vi "test Print Entry with Sub-Entries.vi"(11 "Test Case In":refnum<class "test Electronic Datasheet.lvclass">) -> (0 "error out":errorcluster, 3 "Test Case Out":refnum<class "test Electronic Datasheet.lvclass">)   [LabVIEW 2024, in "test Electronic Datasheet.lvclass"]
uses:
  test Electronic Datasheet.lvclass
  C:/Program Files/National Instruments/LabVIEW 2024/vi.lib/Astemes/LUnit/Test Case.lvclass
  <vilib>/Astemes/LUnit/Test Case.lvclass/Test Case.ctl
  2aee4a49-973f-4d4e-9175-22173d17c8e6.vi
  <vilib>/Astemes/LUnit/Append Pass Result.vi
  <vilib>/Astemes/LUnit/Append Fail Result.vi
  <vilib>/Astemes/LUnit/Describe Comparison.vi
  2aee4a49-973f-4d4e-9175-22173d17c8e6.vi/9c5d11cd-9439-4240-a1ee-d9baace9c924.vi
  <vilib>/Astemes/LUnit/Run In UI.vi
  <vilib>/Utility/error.llb/Clear Errors.vi
  Electronic Datasheet/utils/Electronic Datasheet_GetAttributes.vi
  <vilib>/Astemes/LUnit/Describe Variant.vi
  Electronic Datasheet/Electronic Datasheet.lvclass
  Core/OD Entry/OD Entry.lvclass
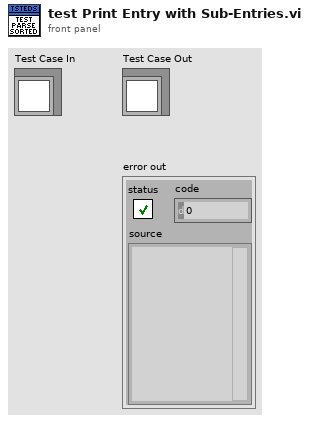
[diagram p1: front panel]
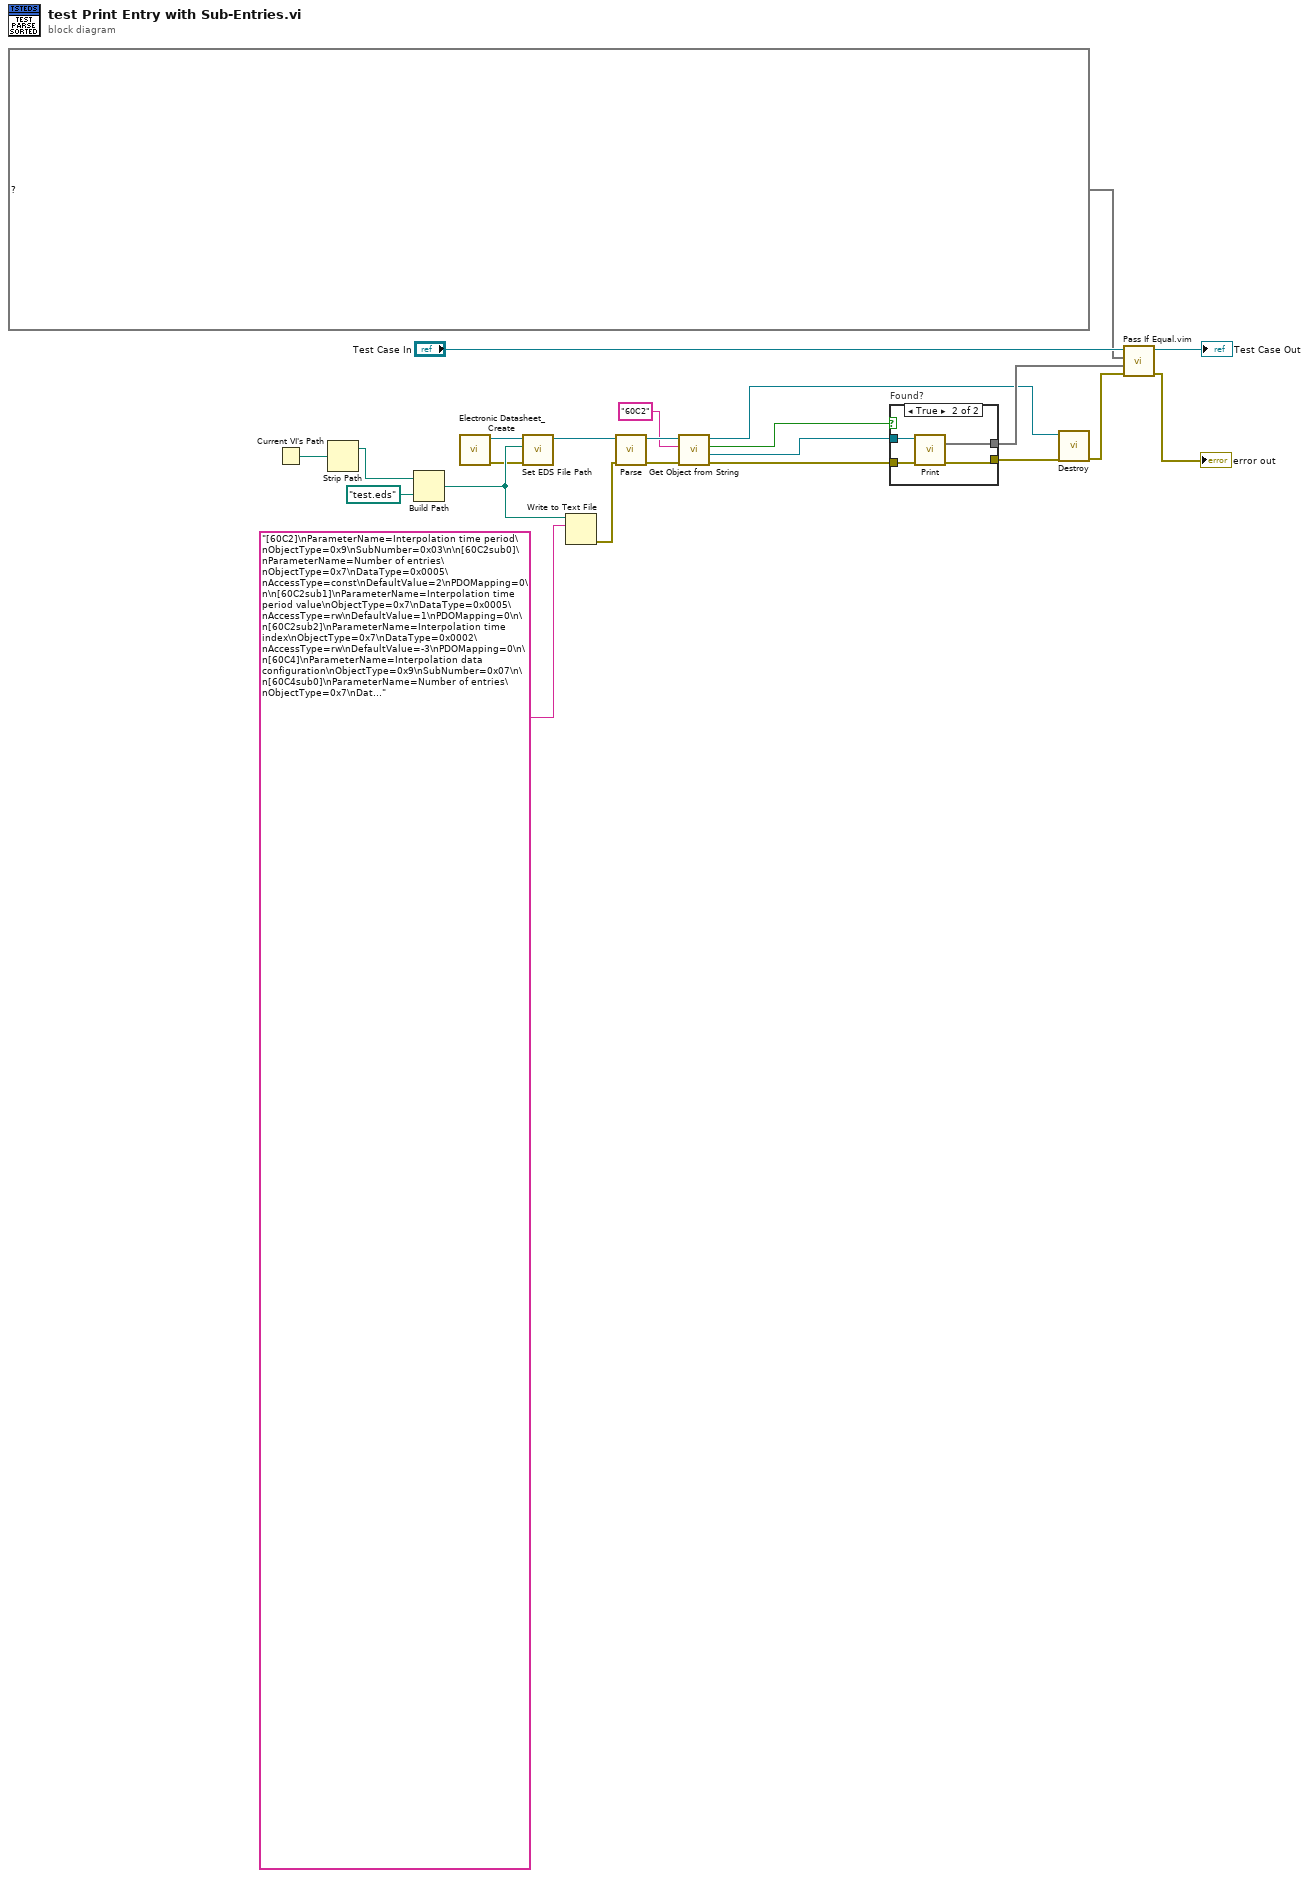
[diagram p0: block diagram]
diagram:
  n1 = Current VI's Path() -> (path=w19:path)
  n2 = Strip Path(path=w19) -> (stripped path=w15:path)  [unwired: 1 out]
  n3 = Build Path(base path=w15, name or relative path=path "test.eds") -> (appended path=w16:path)
  n4 = call "Electronic Datasheet_Create.vi"() -> ("Error Out"=w7:errorcluster, "reference out"=w8:refnum<class "Electronic Datasheet.lvclass">)  [unwired: 10 in]
  n5 = call "Set EDS File Path.vi"("error in"=w7, "EDS File Path"=w16, "reference in"=w8) -> ("reference out"=w20:refnum<class "Electronic Datasheet.lvclass">)  [unwired: 7 in, 1 out]
  n6 = Write to Text File(file (use dialog)=w16, text="[60C2]\nParameterName=Interpolation time period\nObjectType=0x9\nSubNumber=0x03\n\n[60C2sub0]\nParameterName=Number of entries\nObjectType=0x7\nDataType=0x0005\nAccessType=const\nDefaultValue=2\nPDOMapping=0\n\n[60C2sub1]\nParameterName=Interpolation time period value\nObjectType=0x7\nDataType=0x0005\nAccessType=rw\nDefaultValue=1\nPDOMapping=0\n\n[60C2sub2]\nParameterName=Interpolation time index\nObjectType=0x7\nDataType=0x0002\nAccessType=rw\nDefaultValue=-3\nPDOMapping=0\n\n[60C4]\nParameterName=Interpolation data configuration\nObjectType=0x9\nSubNumber=0x07\n\n[60C4sub0]\nParameterName=Number of entries\nObjectType=0x7\nDataType=0x0005\nAccessType=const\nDefaultValue=6\nPDOMapping=0\n\n[60C4sub1]\nParameterName=MaximumBufferSize\nObjectType=0x7\nDataType=0x0007\nAccessType=ro\nDefaultValue=1\nPDOMapping=0\n\n[60C4sub2]\nParameterName=ActualBufferSize\nObjectType=0x7\nDataType=0x0007\nAccessType=rw\nDefaultValue=1\nPDOMapping=0\n\n[60C4sub3]\nParameterName=BufferOrganization\nObjectType=0x7\nDataType=0x0005\nAccessType=rw\nDefaultValue=0\nPDOMapping=0\n\n[60C4sub4]\nParameterName=BufferPosition\nObjectType=0x7\nDataType=0x0006\nAccessType=rw\nDefaultValue=1\nPDOMapping=0\n\n[60C4sub5]\nParameterName=SizeOfDataRecord\nObjectType=0x7\nDataType=0x0005\nAccessType=wo\nDefaultValue=4\nPDOMapping=0\n\n[60C4sub6]\nParameterName=BufferClear\nObjectType=0x7\nDataType=0x0005\nAccessType=wo\nDefaultValue=0\nPDOMapping=0") -> (error out=w17:errorcluster)  [unwired: 2 in, 2 out]
  n7 = call "Parse.vi"("error in"=w17, "reference in"=w20) -> ("error out"=w11:errorcluster, "reference out"=w5:refnum<class "Electronic Datasheet.lvclass">)  [unwired: 8 in]
  n8 = call "Get Object from String.vi"("error in"=w11, "Index"="60C2", "reference in"=w5) -> ("error out"=w6:errorcluster, "OD Entry"=w2:refnum<class "OD Entry.lvclass">, "Found?"=w1:bool, "reference out"=w3:refnum<class "Electronic Datasheet.lvclass">)  [unwired: 5 in]
  n9 = case "Found?" shown="True" w1 {
    tunnel: w2 -> [_ w28]
    tunnel: w6 -> [w24 w27]
    tunnel: [w24 w26] -> w12
    tunnel: [_ w25] -> w10
    frame False {
    }
    frame True {
      n10 = call "Print.vi"("error in"=w27, "OD Entry in"=w28) -> ("error out"=w26:errorcluster, "Entry with Sub-Entries"=w25:map{string, string}[])  [unwired: 7 in, 1 out]
    }
  }
  n11 = call-dynamic "Destroy.vi"("Error In"=w12, "reference in"=w3) -> ("Error Out"=w13:errorcluster)  [unwired: 8 in, 1 out]
  n12 = call "Pass If Equal.vim"("error in (no error)"=w13, "Actual"=w10, "Expected"=map{string, string}[] [{"AccessType"="const", "CompactSubObj"="0", "DataType"="", "DefaultValue"="", "HighLimit"="", "Index"="0x60C2", "LowLimit"="", "ObjFlags"="0", "ObjectType"="RECORD", "PDOMapping"="0", "ParameterName"="Interpolation time period", "SubNumber"="3"}, {"AccessType"="const", "CompactSubObj"="0", "DataType"="UNSIGNED8", "DefaultValue"="2", "HighLimit"="", "Index"="0x00", "LowLimit"="", "ObjFlags"="0", "ObjectType"="VAR", "PDOMapping"="0", "ParameterName"="Number of entries", "SubNumber"=""}, {"AccessType"="rw", "CompactSubObj"="0", "DataType"="UNSIGNED8", "DefaultValue"="1", "HighLimit"="", "Index"="0x01", "LowLimit"="", "ObjFlags"="0", "ObjectType"="VAR", "PDOMapping"="0", "ParameterName"="Interpolation time period value", "SubNumber"=""}, {"AccessType"="rw", "CompactSubObj"="0", "DataType"="INTEGER8", "DefaultValue"="-3", "HighLimit"="", "Index"="0x02", "LowLimit"="", "ObjFlags"="0", "ObjectType"="VAR", "PDOMapping"="0", "ParameterName"="Interpolation time index", "SubNumber"=""}] ("Entry with Sub-Entries"), "LUnit Test Case In"="Test Case In") -> ("error out"=→"error out":errorcluster, "LUnit Test Case Out"=→"Test Case Out":refnum<class "test Electronic Datasheet.lvclass">)  [unwired: 6 in]
